vi "RabbitMQExample.vi"   [LabVIEW 2019]
uses:
  API/config.ctl
  rabbitmq.lvlib
types:
  T1 = typedef "rabbitmq.lvlib/config.ctl" = cluster{"host":string, "port":i32, "virtual_host":string, "username":string, "password":string}
  T2 = typedef "rabbitmq.lvlib/session.ctl" = cluster{"script_path":path, "python_session":refnum<k35>}
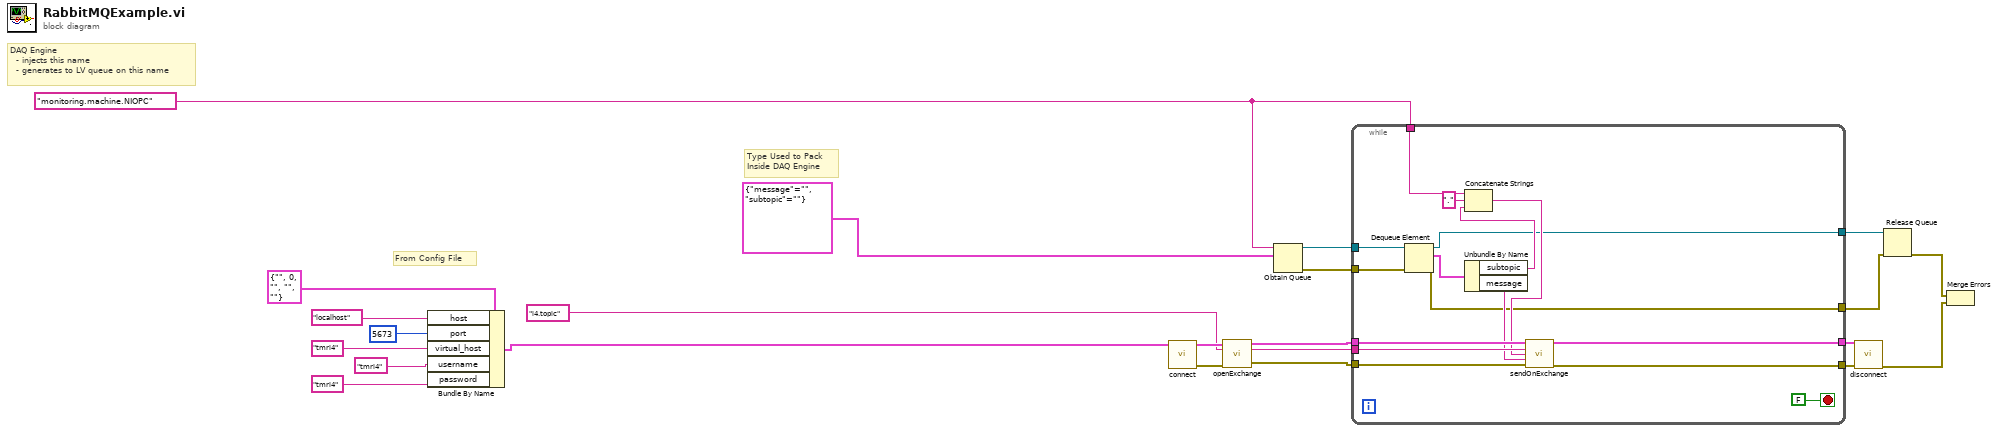
[diagram p0: block diagram]
diagram:
  w9 = "monitoring.machine.NIOPC"
  # "Type Used to Pack \nInside DAQ Engine"
  # "From Config File"
  # "DAQ Engine \n  - injects this name\n  - generates to LV queue on this name"
  n1 = Bundle By Name(cluster=T1 {"host"="", "port"=0, "virtual_host"="", "username"="", "password"=""} ("Cluster"), "host"="localhost", "port"=5673, "virtual_host"="tmri4", "username"="tmri4", "password"="tmri4") -> (w15:T1)
  n2 = call "connect.vi"("RabbitMQ Config"=w15) -> ("error out"=w5:errorcluster, "RabbitMQ Session Out"=w4:T2)  [unwired: 9 in]
  n3 = call "openExchange.vi"("error in (no error)"=w5, "Exchange Name In"="i4.topic", "RabbitMQ Session In"=w4) -> ("error out"=w13:errorcluster, "Exchange Name out"=w12:string, "RabbitMQ Session Out"=w14:T2)  [unwired: 6 in]
  n4 = Obtain Queue(name (unnamed)=w9, element data type=cluster{"message":string, "subtopic":string} {"message"="", "subtopic"=""}) -> (queue out=w10:refnum<queue>, error out=w7:errorcluster)  [unwired: 3 in, 1 out]
  n5 = while {
    tunnel: [w39] -> w17
    tunnel: [w38] -> w16
    tunnel: w14 -> [w37]
    tunnel: w13 -> [w36]
    tunnel: w12 -> [w35]
    tunnel: w10 -> [w32]
    tunnel: w9 -> [w31]
    tunnel: [w27] -> w8
    tunnel: w7 -> [w26]
    tunnel: [w25] -> w6
    stop <- FALSE stop-if-true
    n6 = Dequeue Element(queue=w32, error in (no error)=w26) -> (queue out=w27:refnum<queue>, element=w33:cluster{"message":string, "subtopic":string}, error out=w25:errorcluster)  [unwired: 1 in, 1 out]
    n7 = Unbundle By Name(w33) -> ("subtopic"=w34:string, "message"=w29:string)
    n8 = Concatenate Strings(w31, "." ("string"), w34) -> (w28:string)
    n9 = call "sendOnExchange.vi"("RabbitMQ Session In"=w37, "Exchange Name in"=w35, "Routing Key in"=w28, "Message In"=w29, "error in (no error)"=w36) -> ("RabbitMQ Session Out"=w38:T2, "error out"=w39:errorcluster)  [unwired: 6 in, 3 out]
  }
  n10 = call "disconnect.vi"("error in (no error)"=w17, "RabbitMQ Session In"=w16) -> ("error out"=w2:errorcluster)  [unwired: 9 in]
  n11 = Release Queue(queue=w8, error in (no error)=w6) -> (error out=w1:errorcluster)  [unwired: 1 in, 2 out]
  n12 = Merge Errors(w1, w2) -> ()  [unwired: 1 out]
